vi "loadcellpractice.vi"() -> ()   [LabVIEW 2014]
panel:
  in  "stop":bool
  out "Voltage":dynamicdata(graph)
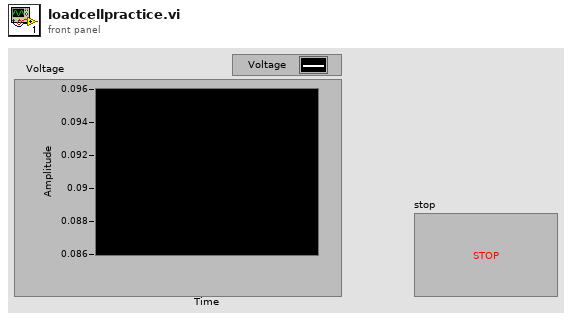
[diagram p1: front panel]
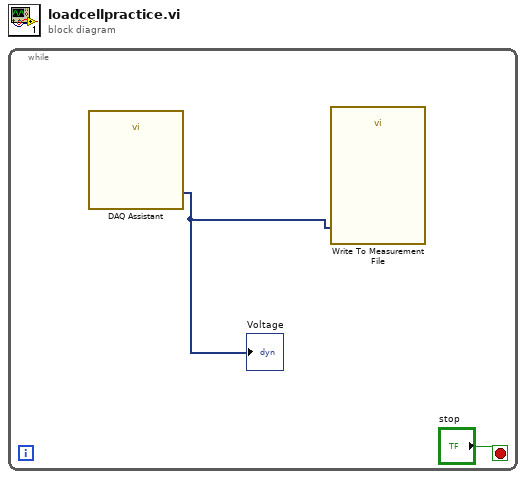
[diagram p0: block diagram]
diagram:
  n1 = while {
    stop <- "stop" stop-if-true
    n2 = call "DAQ Assistant"() -> ("data"=w2:dynamicdata)  [unwired: 17 in, 2 out]
    "Voltage" <- w2
    n3 = call "Write To Measurement File"("Signals"=w2) -> ()  [unwired: 16 in, 3 out]
  }
